vi "GP307 Read-RT.vi"(8 "error in (no error)":errorcluster, 10 "Delay Time (s)":dbl=3.0 format="%#_13g", 11 "VISA Refnum in":refnum<visa-resource-name>) -> (0 "error out":errorcluster, 2 "GP307 output":T1, 3 "VISA Refnum out":refnum<visa-resource-name>)   [LabVIEW 2016]
doc: "Reads both convectrons and ion gauges from a Granville-Phillips 307 Vacuum gauge controller. Gauge controller should be connected via serial cable to cRIO controller. This VI is meant to used in real-time code on cRIO run in Scan-Engine mode."
uses:
  Controls/GP307 cluster.ctl
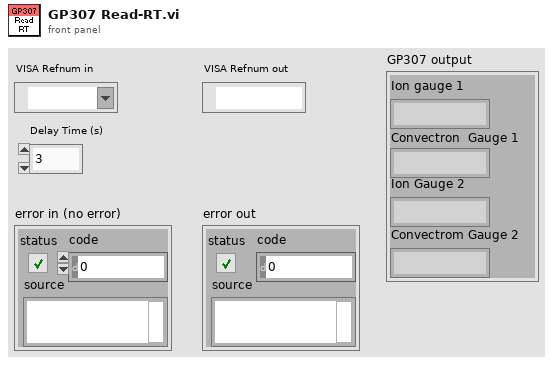
[diagram p1: front panel]
types:
  T1 = typedef "GP307 cluster.ctl" = cluster{"Ion gauge 1":string, "Convectron  Gauge 1 ":string, "Ion Gauge 2":string, "Convectrom Gauge 2":string}
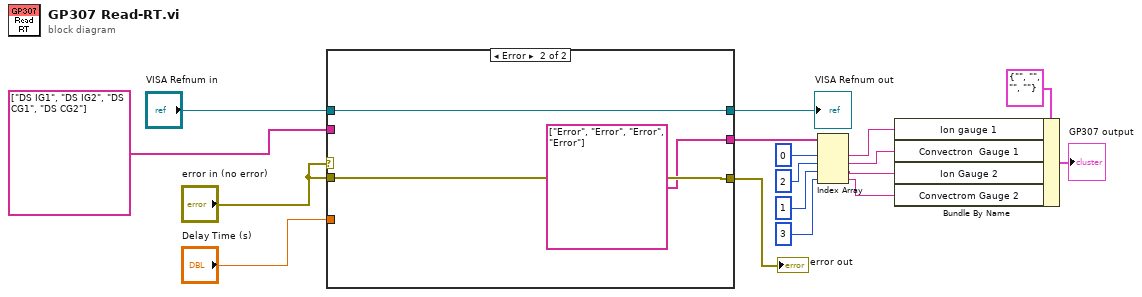
[diagram p0: block diagram]
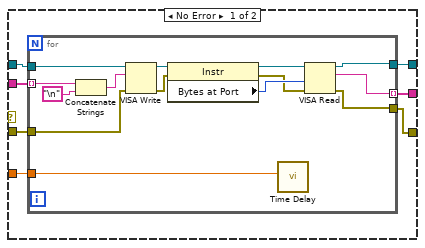
[diagram p2: hidden frame]
diagram:
  n1 = case shown="Error" "error in (no error)" {
    tunnel: "Delay Time (s)" -> [w24 _]
    tunnel: string[] ["DS IG1", "DS IG2", "DS CG1", "DS CG2"] -> [w23 _]
    tunnel: [w22 w40] -> w15
    tunnel: "error in (no error)" -> [w21 w40]
    tunnel: [w20 string[] ["Error", "Error", "Error", "Error"]] -> w6
    tunnel: [w19 w41] -> w14
    tunnel: "VISA Refnum in" -> [w18 w41]
    frame No Error {
      n2 = for {
        tunnel: w23 -> [w33] mode=indexing
        tunnel: w18 -> [w32]
        tunnel: [w31] -> w19
        tunnel: [w25] -> w20 mode=indexing
        tunnel: w21 -> [w30]
        tunnel: [w27] -> w22
        tunnel: w24 -> [w26]
        n3 = Concatenate Strings(w33, "\n") -> (w34:string)
        n4 = VISA Write(VISA resource name=w32, write buffer=w34, error in (no error)=w30) -> (VISA resource name out=w38:refnum<visa-resource-name>, error out=w29:errorcluster)  [unwired: 1 out]
        n5 = property class="Instr"(reference=w38, error in=w29) -> (reference out=w37:refnum<visa-resource-name>, error out=w28:errorcluster, "Bytes at Port"=w35:u32)
        n6 = call "Time Delay"("Delay Time (s)"=w26) -> ()  [unwired: 10 in, 1 out]
        n7 = VISA Read(VISA resource name=w37, byte count=w35, error in (no error)=w28) -> (VISA resource name out=w31:refnum<visa-resource-name>, read buffer=w25:string, error out=w27:errorcluster)  [unwired: 1 out]
      }
    }
    frame Error {
    }
  }
  "error out" <- w15
  "VISA Refnum out" <- w14
  n8 = Index Array(array=w6, index #1=0 ("index"), index #2=2 ("index"), index #3=1 ("index"), index #4=3 ("index")) -> (element #1=w5:string, element #2=w4:string, element #3=w3:string, element #4=w2:string)
  n9 = Bundle By Name(cluster=T1 {"Ion gauge 1"="", "Convectron  Gauge 1 "="", "Ion Gauge 2"="", "Convectrom Gauge 2"=""} ("Vac gauge cluster control"), "Ion gauge 1"=w5, "Convectron  Gauge 1"=w4, "Ion Gauge 2"=w3, "Convectrom Gauge 2"=w2) -> (→"GP307 output":T1)
